vi "Configure BrowerTree Icon.vi"(8 "error in (no error)":errorcluster, 11 "BrowerTree in":refnum<class "BrowerTree.lvclass">) -> (0 "error out":errorcluster, 3 "BrowerTree out":refnum<class "BrowerTree.lvclass">)   [LabVIEW 2015, in "BrowerTree.lvclass"]
uses:
  BrowerTree.lvclass
  BrowerTree.lvclass/BrowerTree.ctl
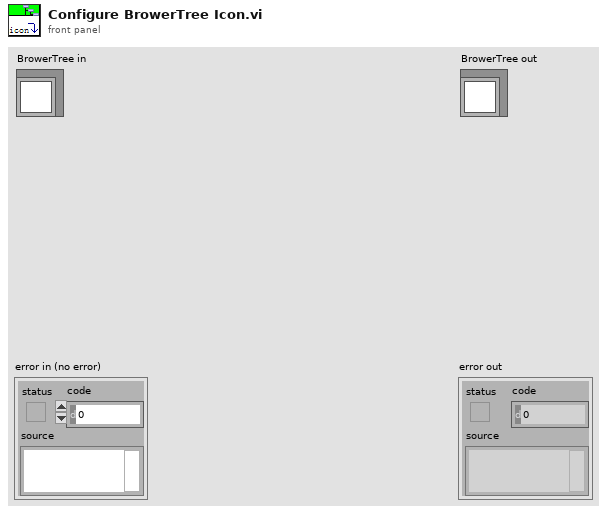
[diagram p1: front panel]
types:
  T1 = typedef "imagedata.ctl" = cluster{"image type":i32, "image depth":i32, "image":u8[], "mask":u8[], "colors":u32[], "Rectangle":cluster{"left":i16, "top":i16, "right":i16, "bottom":i16}}
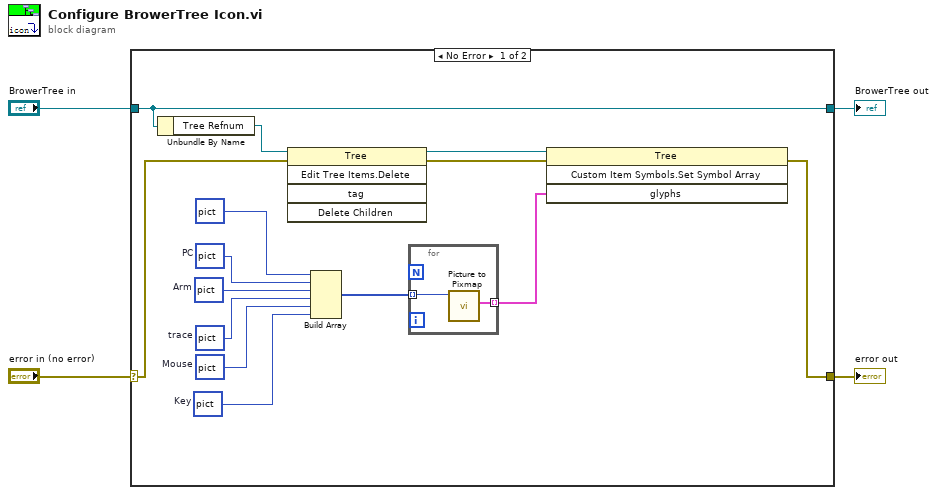
[diagram p0: block diagram]
diagram:
  n1 = case shown="No Error" "error in (no error)" {
    selector: "error in (no error)" -> [w7 w22]
    tunnel: [w5 w22] -> w3
    tunnel: [w18 w21] -> w1
    tunnel: "BrowerTree in" -> [w18 w21]
    frame No Error {
      w13 = picture bytes[830]  # Arm
      w12 = picture bytes[830]  # trace
      w14 = picture bytes[830]  # PC
      w10 = picture bytes[830]  # Key
      w11 = picture bytes[830]  # Mouse
      n2 = Unbundle By Name(w18) -> ("Tree Refnum"=w17:refnum<vi>)
      n3 = invoke class="Tree" method="Edit Tree Items.Delete"(reference=w17, error in=w7) -> (reference out=w16:refnum<vi>, error out=w6:errorcluster)  [unwired: 3 in, 3 out]
      n4 = Build Array(picture data[5B] ("2D Picture"), w14, w13, w12, w11, w10) -> (w9:picture[])
      n5 = for {
        tunnel: [w20] -> w8 mode=indexing
        tunnel: w9 -> [w19] mode=indexing
        n6 = call <vilib>:"Picture to Pixmap.vi"("picture"=w19) -> ("image data"=w20:T1)  [unwired: 9 in, 1 out]
      }
      n7 = invoke class="Tree" method="Custom Item Symbols.Set Symbol Array"(reference=w16, error in=w6, "glyphs"=w8) -> (error out=w5:errorcluster)  [unwired: 1 in, 3 out]
    }
    frame Error {
    }
  }
  "error out" <- w3
  "BrowerTree out" <- w1
